vi "SENS_CORR_EXT_AUTO_CONF.vi"(0 "VISA IN":refnum<visa-resource-name>, 1 "Frequencies":string, 5 "error in":errorcluster, 7 "Channel":i32) -> (14 "VISA Out":refnum<visa-resource-name>, 19 "error out":errorcluster)   [LabVIEW 2018, in "PNA-X.lvlib"]
doc: "SENSe<cnum>:CORRection:EXTension:AUTO:CONFig <char> \n(Read-Write) Sets the frequencies used to calculate Automatic Port Extension. Learn more about \ncalculating Automatic Port Extension. \nParameters \n<cnum> Any existing channel number. If unspecified, value is set to 1 \n<char> Frequencies to be used: \nCSPN Use current frequency span. \nAMKR - Use active marker frequency. \nUSPN - Use custom user span. Use SENS:CORR:EXT:AUTO:STAR and \nSENS:CORR:EXT:AUTO:STOP to specify start and stop frequency. \nExamples SENS:CORR:EXT:AUTO:CONF CSPN \nsense2:correction:extension:auto:config amkr \nQuery Syntax SENSe<cnum>:CORRection:EXTension:AUTO:CONFig ? \n1700\n\nReturn Type Character \nDefault CSPN"
uses:
  PNA-X.lvlib
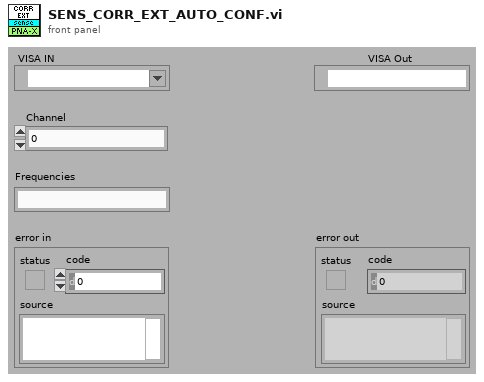
[diagram p1: front panel]
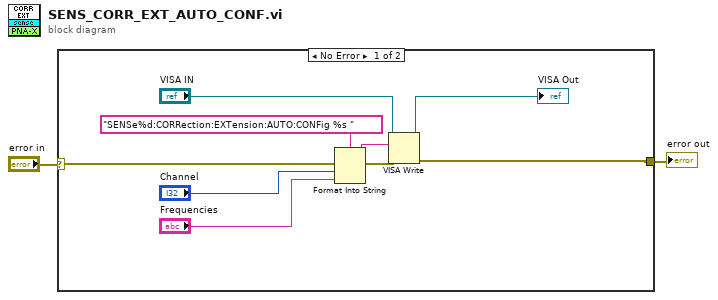
[diagram p0: block diagram]
diagram:
  n1 = case shown="No Error" "error in" {
    selector: "error in" -> [w11 w12]
    tunnel: [w6 w12] -> w1
    frame No Error {
      n2 = Format Into String(format string="SENSe%d:CORRection:EXTension:AUTO:CONFig %s " ("Cmdline"), error in=w11, "Channel", "Frequencies") -> (resulting string=w9:string, error out=w10:errorcluster)  [unwired: 1 in]
      n3 = VISA Write(VISA resource name="VISA IN", write buffer=w9, error in (no error)=w10) -> (VISA resource name out=→"VISA Out":refnum<visa-resource-name>, error out=w6:errorcluster)  [unwired: 1 out]
    }
    frame Error {
    }
  }
  "error out" <- w1
